vi "meta_readFileBlock.vi"(8 "error in (no error)":errorcluster, 11 "meta file in":T1) -> (0 "error out":errorcluster, 2 "file info":T4, 3 "meta file out":T1)   [LabVIEW 2017, in "NI_ExcelFile.lvlib"]
uses:
  <vilib>/express/express shared/NI_ExcelFile/NI_ExcelFile.lvlib
  <vilib>/express/express shared/NI_ExcelFile/Ctrls/meta_FileInfo.ctl
  <vilib>/express/express shared/NI_ExcelFile/Ctrls/meta_FileInfo_2013.ctl
  <vilib>/express/express shared/NI_ExcelFile/Ctrls/FileAttribute.ctl
  <vilib>/express/express shared/NI_ExcelFile/Ctrls/meta_file.ctl
  <vilib>/express/express shared/NI_ExcelFile/Ctrls/meta_Block.ctl
  <vilib>/express/express shared/NI_ExcelFile/Ctrls/meta_BlockType.ctl
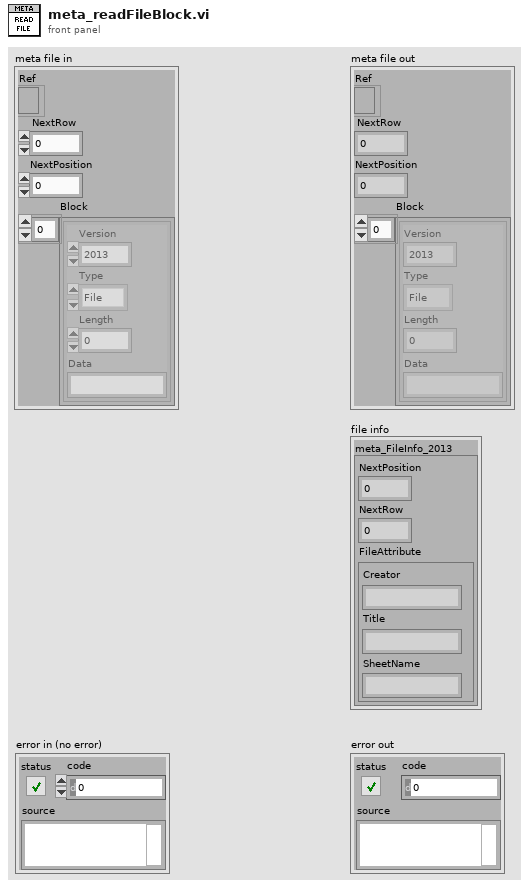
[diagram p1: front panel]
types:
  T1 = typedef "NI_ExcelFile.lvlib/meta_file.ctl" = cluster{"Ref":refnum<file>, "NextRow":i32, "NextPosition":i64, "Block":T2[]}
  T2 = typedef "NI_ExcelFile.lvlib/meta_Block.ctl" = cluster{"Version":u16, "Type":T3, "Length":i32, "Data":string}
  T3 = typedef "NI_ExcelFile.lvlib/meta_BlockType.ctl" = enum16{"NITag", "File", "Column"}
  T4 = typedef "NI_ExcelFile.lvlib/meta_FileInfo.ctl" = cluster{"meta_FileInfo_2013":T5}
  T5 = typedef "NI_ExcelFile.lvlib/meta_FileInfo_2013.ctl" = cluster{"NextPosition":i64, "NextRow":i32, "FileAttribute ":T6}
  T6 = typedef "NI_ExcelFile.lvlib/FileAttribute.ctl" = cluster{"Creator":string, "Title":string, "SheetName":string}
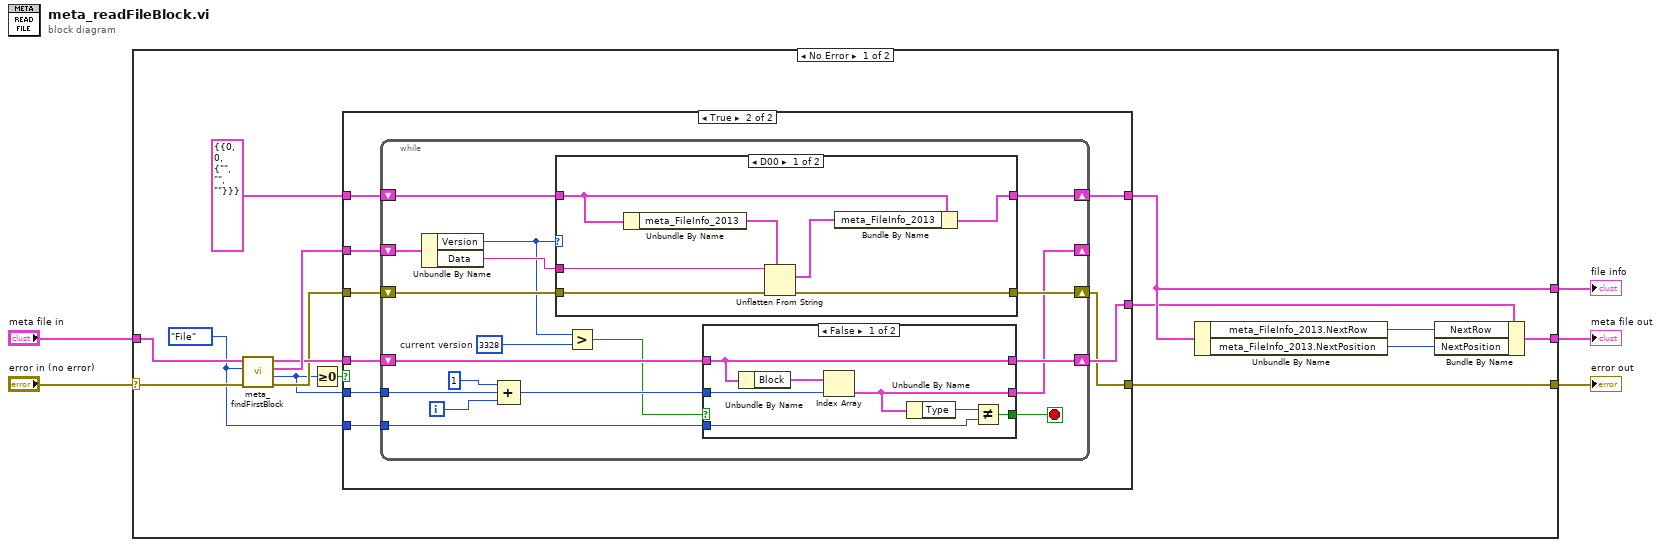
[diagram p0: block diagram]
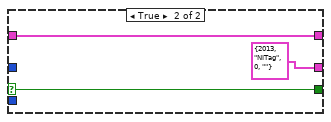
[diagram p3: hidden frame]
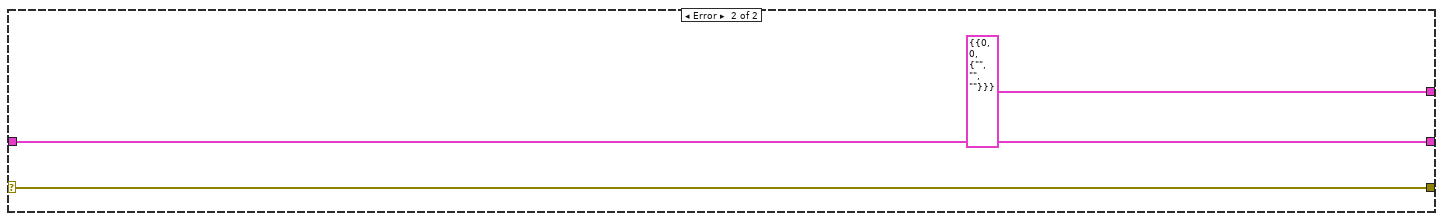
[diagram p5: hidden frame]
diagram:
  n1 = case shown="No Error" "error in (no error)" {
    selector: "error in (no error)" -> [w16 w70]
    tunnel: [w20 w72] -> w5
    tunnel: "meta file in" -> [w19 w72]
    tunnel: [w9 w70] -> w3
    tunnel: [w11 T4 {"meta_FileInfo_2013"={"NextPosition"=0, "NextRow"=0, "FileAttribute "={"Creator"="", "Title"="", "SheetName"=""}}} ("meta_FileInfo")] -> w2
    frame No Error {
      w6 = meta_BlockType."File" ("block type")
      n2 = call <vilib>:"meta_findFirstBlock.vi"("error in"=w16, "block type"=w6, "meta file in"=w19) -> ("error out"=w8:errorcluster, "index"=w7:i32, "block out"=w14:T2, "meta file out"=w12:T1)  [unwired: 5 in]
      n3 = Greater Or Equal To 0?(x=w7) -> (x >= 0?=w15:bool)
      n4 = case shown="True" w15 {
        tunnel: w14 -> [_ w32]
        tunnel: T4 {"meta_FileInfo_2013"={"NextPosition"=0, "NextRow"=0, "FileAttribute "={"Creator"="", "Title"="", "SheetName"=""}}} ("meta_FileInfo") -> [w22 w31]
        tunnel: w8 -> [w23 w30]
        tunnel: w12 -> [w21 w29]
        tunnel: [w22 w28] -> w11
        tunnel: [w21 w27] -> w10
        tunnel: [w23 w26] -> w9
        tunnel: w7 -> [_ w25]
        tunnel: w6 -> [_ w24]
        frame False {
        }
        frame True {
          n5 = while {
            shift-right: [w42] -> _
            shift-left: w32 -> [w50]
            shift-right: [w47] -> w28
            shift-left: w31 -> [w48]
            shift-right: [w45] -> w26
            shift-left: w30 -> [w46]
            shift-right: [w43] -> w27
            shift-left: w29 -> [w44]
            tunnel: w25 -> [w40]
            tunnel: w24 -> [w33]
            i -> [w38]
            stop <- w34 stop-if-true
            w36 = u16 3328  # current version
            n6 = Unbundle By Name(w50) -> ("Version"=w41:u16, "Data"=w49:string)
            n7 = Compound Arithmetic op=ADD(1 ("value"), w40, w38) -> (w39:i32)
            n8 = case shown="D00" w41 {
              tunnel: w49 -> [w65 _]
              tunnel: w48 -> [w66 w69]
              tunnel: [w67 w69] -> w47
              tunnel: w46 -> [w62 w68]
              tunnel: [w61 w68] -> w45
              frame 3328 {
                n9 = Unbundle By Name(w66) -> ("meta_FileInfo_2013"=w64:T5)
                n10 = Unflatten From String(type=w64, binary string=w65, error in (no error)=w62) -> (value=w63:T5, error out=w61:errorcluster)  [unwired: 2 in, 1 out]
                n11 = Bundle By Name(cluster=w66, "meta_FileInfo_2013"=w63) -> (w67:T4)
              }
              frame Default {
              }
            }
            n12 = Greater?(x=w41, y=w36) -> (0:w35:bool)
            n13 = case shown="False" w35 {
              selector: w35 -> [_ w58]
              tunnel: w44 -> [w55 w60]
              tunnel: w39 -> [w57 _]
              tunnel: [w55 w60] -> w43
              tunnel: [w54 T2 {"Version"=2013, "Type"=enum."NITag", "Length"=0, "Data"=""} ("Block")] -> w42
              tunnel: [w53 w58] -> w34
              tunnel: w33 -> [w51 _]
              frame False {
                n14 = Unbundle By Name(w55) -> ("Block"=w56:T2[])
                n15 = Index Array(array=w56, index=w57) -> (element=w54:T2)
                n16 = Unbundle By Name(w54) -> ("Type"=w52:T3)
                n17 = Not Equal?(x=w52, y=w51) -> (x != y?=w53:bool)
              }
              frame True {
              }
            }
          }
        }
      }
      n18 = Unbundle By Name(w11) -> ("meta_FileInfo_2013.NextRow"=w17:i32, "meta_FileInfo_2013.NextPosition"=w18:i64)
      n19 = Bundle By Name(cluster=w10, "NextRow"=w17, "NextPosition"=w18) -> (w20:T1)
    }
    frame Error {
    }
  }
  "meta file out" <- w5
  "error out" <- w3
  "file info" <- w2
